vi "realtime_trans.vi"() -> ()   [LabVIEW 2015]
uses:
  <vilib>/rvi/interface/nirviOpenFPGA/nirviOpenFPGA.xnode
  <vilib>/rvi/interface/nirviReadWriteControl/nirviReadWriteControl.xnode
  <vilib>/Instr/_visa.llb/VISA Configure Serial Port (Instr).vi
  FPGA/FPGA_Transmission.vi
  <vilib>/functionblocks/FB Core/FB Core.xnode
  <vilib>/functionblocks/Control/PID/PID.vi
  <vilib>/functionblocks/NI_FunctionBlock Libraries.lvlib
  NiFpgaLv.dll
  <vilib>/Utility/error.llb/Error Cluster From Error Code.vi
  <vilib>/rvi/errors/niLvFpgaAdjustHostInterfaceError.vi
  FPGA Bitfiles/Controlsoftware2_FPGATarget4_FPGATransmission_apjjT0zB-SU.lvbitx
  <vilib>/FPGAPlugInAG/cRIO-9074/niLvFpga_Open_cRIO-9074.vi
panel:
  in  "Tab Control":enum32{"control", "Junk"}(tab)
  out "Steerer X+":dbl
  out "Steerer X-":dbl
  out "Steerer Y+":dbl
  out "Steerer Y-":dbl
  out "ExB +":dbl
  out "ExB -":dbl
  out "X+ V":fxp<+/-,26,5> format="%.23g"
  out "X+ I":fxp<+/-,26,5> format="%_4g"
  out "X- V":fxp<+/-,26,5> format="%_4g"
  out "X-I":fxp<+/-,26,5> format="%_4g"
  out "Y+ V":fxp<+/-,26,5> format="%_4g"
  out "Y+I":fxp<+/-,26,5> format="%_4g"
  out "Y-V":fxp<+/-,26,5> format="%_4g"
  out "Y-I":fxp<+/-,26,5> format="%_4g"
  out "ExB + V":fxp<+/-,26,5> format="%_4g"
  out "ExB +I":fxp<+/-,26,5> format="%_4g"
  out "ExB -V":fxp<+/-,26,5> format="%_4g"
  out "ExB-I":fxp<+/-,26,5> format="%_4g"
  out "concatenated string":string
  out "Ion gauge switch object cluser 2":T1
  out "Ion gauge anal waist Cluster 1":T1
  out "EXB":dbl
  in  "derivative time (Td, min)":dbl=0.05
  in  "integral time (Ti, min)":dbl=0.01
  in  "proportional gain (Kc)":dbl=25.0
  out "concatenated string 2":string
  out "anal field read":dbl
  out "unsigned byte array":u8[](array[numeric])
  out "Analyze read":u8[](array[numeric])
  out "analyze magnet set field":dbl
  out "element":dbl
  in  "diverter":bool
  out "diverter":bool
  out "error out":errorcluster
  out "error out 3":errorcluster
  out "error out 2":errorcluster
  in  "Ion gauge cluster control":T1
  out "Convectron 3":u8[](array[numeric])
  out "Ion gauge 4":u8[](array[numeric])
  out "Convectron 4":u8[](array[numeric])
  out "Ion gauge 5":u8[](array[numeric])
  out "Convectron 2":u8[](array[numeric])
  out "Ion gauge 2":u8[](array[numeric])
  out "Convectron 1":u8[](array[numeric])
  out "Ion gauge 1":u8[](array[numeric])
  out "error out 4":errorcluster
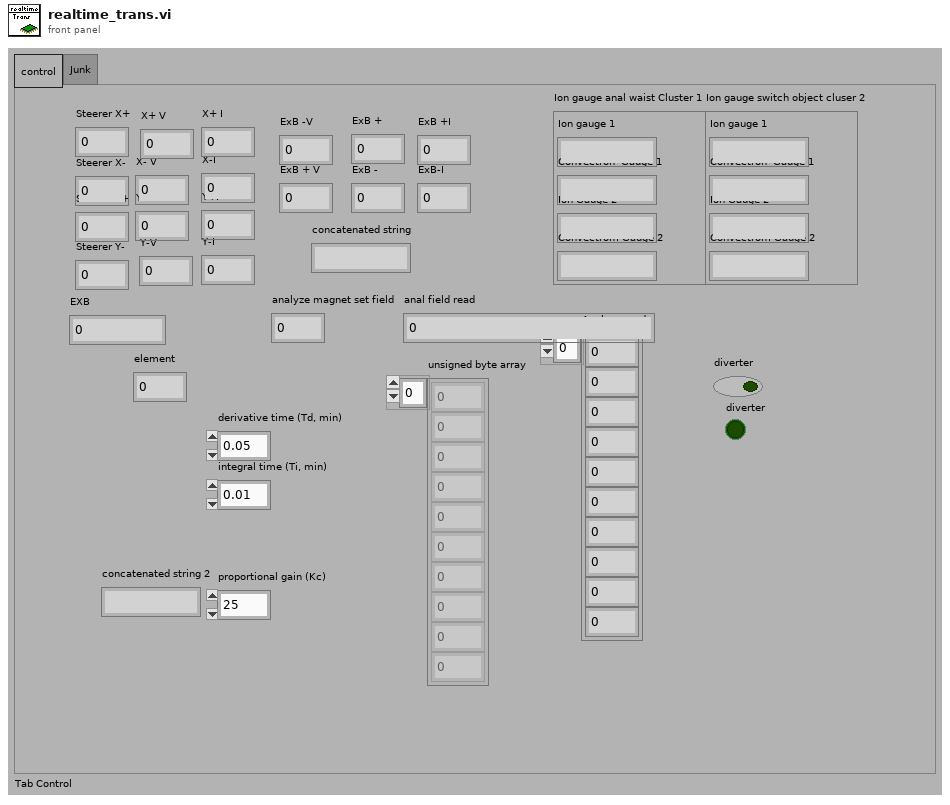
[diagram p1: front panel]
types:
  T1 = cluster{"Ion gauge 1":string, "Convectron  Gauge 1 ":string, "Ion Gauge 2":string, "Convectrom Gauge 2":string}
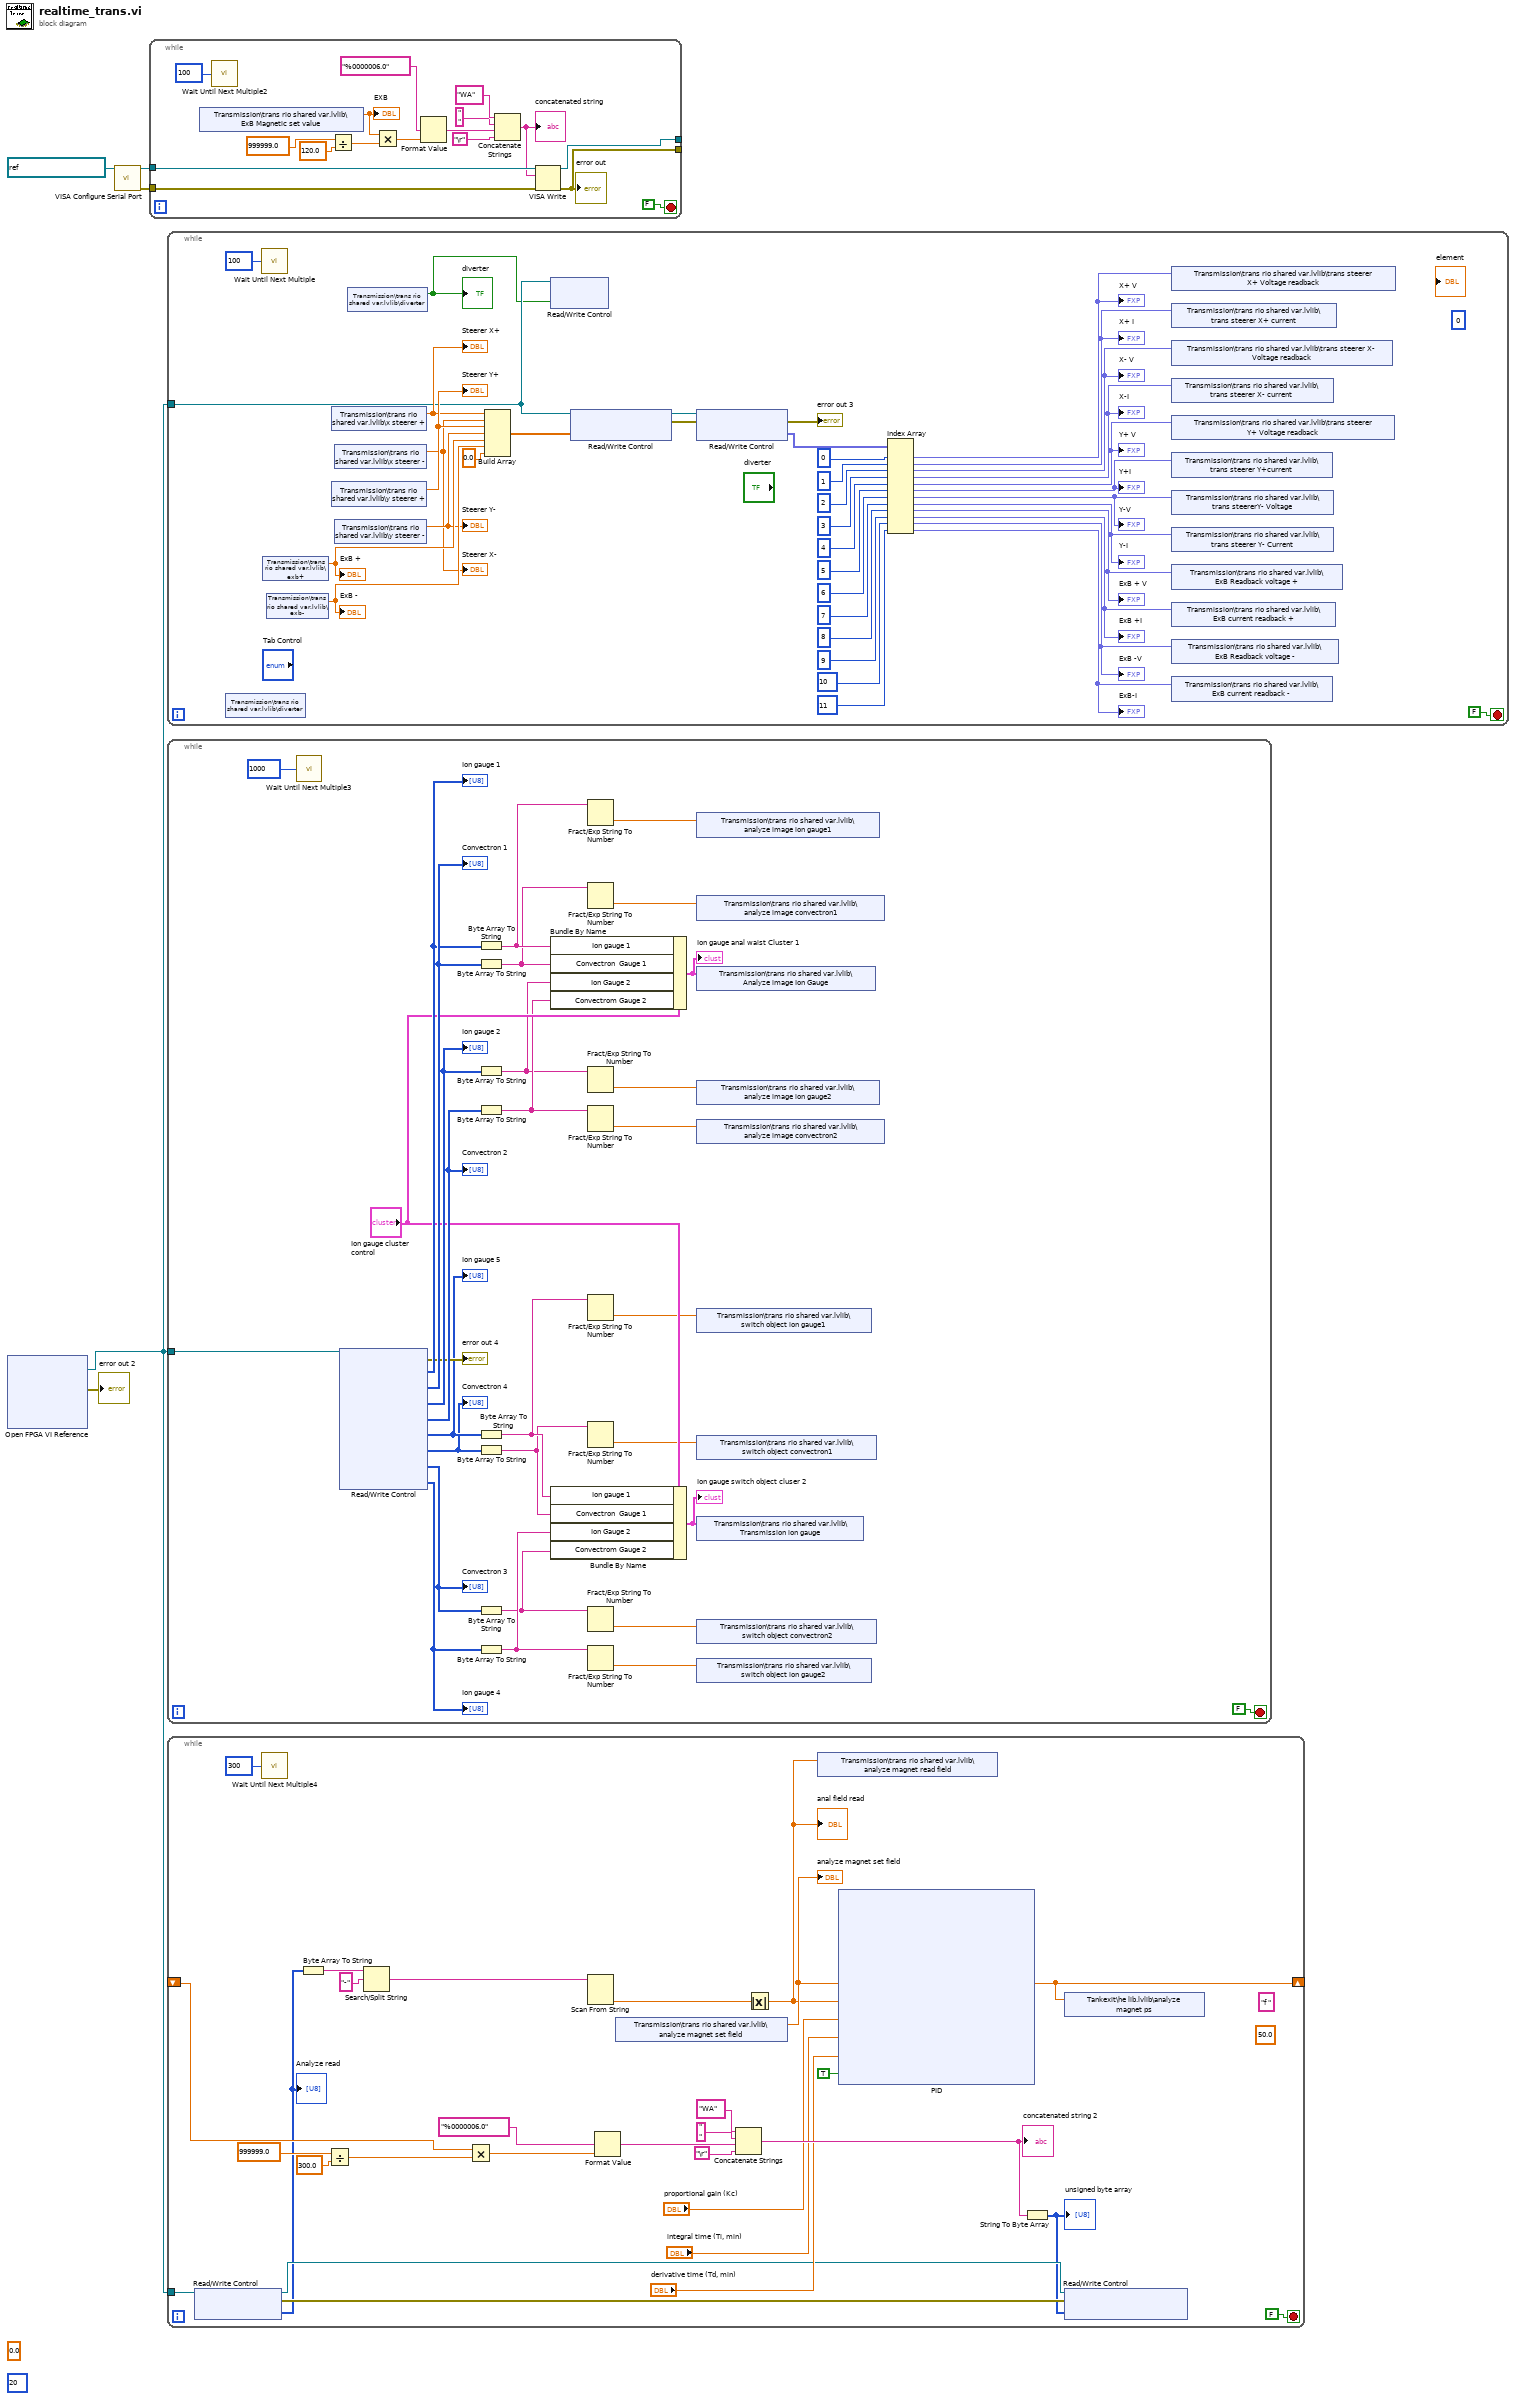
[diagram p0: block diagram]
diagram:
  (unwired) 20 ("dimension size")
  (unwired) 0.0 ("output")
  n1 = xnode "Open FPGA VI Reference"() -> ("FPGA VI Reference Out"=w1:refnum<k20>, "error out"=→"error out 2":errorcluster)  [unwired: 2 in]
  n2 = call-poly "VISA Configure Serial Port"("VISA resource name"=refnum<visa-resource-name> "ASRL1::INSTR") -> ("VISA resource name out"=w5:refnum<visa-resource-name>, "error out"=w4:errorcluster)  [unwired: 5 in, 8 out]
  n3 = while {
    tunnel: w4 -> [w12]
    tunnel: w5 -> [w11]
    tunnel: [w9] -> _
    tunnel: [w8] -> _
    stop <- FALSE stop-if-true
    n4 = shared-variable "Transmission\\trans rio shared var.lvlib\\ExB Magnetic set value"() -> (w7:dbl)  [unwired: 1 in, 1 out]
    "EXB" <- w7
    n5 = call "Wait Until Next Multiple2"("Count(mSec)"=u32 100) -> ()  [unwired: 1 out]
    n6 = Divide(x=999999.0, y=120.0) -> (x/y=w20:dbl)
    n7 = Multiply(x=w7, y=w20) -> (x*y=w13:dbl)
    n8 = Format Value(format string="%0000006.0", value (0)=w13) -> (output string=w16:string)  [unwired: 1 out]
    n9 = Concatenate Strings("WA", " ", w16, "\r") -> (w10:string)
    "concatenated string" <- w10
    n10 = VISA Write(VISA resource name=w11, write buffer=w10, error in (no error)=w12) -> (VISA resource name out=w9:refnum<visa-resource-name>, error out=w8:errorcluster)  [unwired: 1 out]
    "error out" <- w8
  }
  n11 = while {
    tunnel: w1 -> [w24]
    stop <- FALSE stop-if-true
    (unwired) 0 ("dimension size")
    n12 = shared-variable "Transmission\\trans rio shared var.lvlib\\diverter"() -> ()  [unwired: 1 in, 2 out]
    n13 = call "Wait Until Next Multiple"("Count(mSec)"=u32 100) -> ()  [unwired: 1 out]
    n14 = shared-variable "Transmission\\trans rio shared var.lvlib\\exb+"() -> (w47:dbl)  [unwired: 1 in, 1 out]
    "ExB +" <- w47
    n15 = shared-variable "Transmission\\trans rio shared var.lvlib\\exb-"() -> (w48:dbl)  [unwired: 1 in, 1 out]
    "ExB -" <- w48
    n16 = shared-variable "Transmission\\trans rio shared var.lvlib\\x steerer +"() -> (w43:dbl)  [unwired: 1 in, 1 out]
    "Steerer X+" <- w43
    n17 = shared-variable "Transmission\\trans rio shared var.lvlib\\y steerer +"() -> (w45:dbl)  [unwired: 1 in, 1 out]
    "Steerer Y+" <- w45
    n18 = shared-variable "Transmission\\trans rio shared var.lvlib\\x steerer -"() -> (w44:dbl)  [unwired: 1 in, 1 out]
    "Steerer X-" <- w44
    n19 = shared-variable "Transmission\\trans rio shared var.lvlib\\y steerer -"() -> (w46:dbl)  [unwired: 1 in, 1 out]
    "Steerer Y-" <- w46
    n20 = shared-variable "Transmission\\trans rio shared var.lvlib\\diverter"() -> (w23:bool)  [unwired: 1 in, 1 out]
    "diverter" <- w23
    n21 = Build Array(w43, w44, w45, w46, w47, w48, 0.0 ("element")) -> (w62:dbl[])
    n22 = xnode "Read/Write Control"("FPGA VI Reference In"=w24, "diverter"=w23) -> ()  [unwired: 1 in, 2 out]
    n23 = xnode "Read/Write Control"("FPGA VI Reference In"=w24, "Analog Output"=w62) -> ("FPGA VI Reference Out"=w28:refnum<k20>, "error out"=w27:errorcluster)  [unwired: 1 in]
    n24 = xnode "Read/Write Control"("FPGA VI Reference In"=w28, "error in"=w27) -> ("error out"=→"error out 3":errorcluster, "Analog input"=w29:fxp<+/-,26,5>[])  [unwired: 1 out]
    n25 = Index Array(array=w29, index #1=0 ("index"), index #2=1 ("index"), index #3=2 ("index"), index #4=3 ("index"), index #5=4 ("index"), index #6=5 ("index"), index #7=6 ("index"), index #8=7 ("index"), index #9=8 ("index"), index #10=9 ("index"), index #11=10 ("index"), index #12=11 ("index")) -> (element #1=w41:fxp<+/-,26,5>, element #2=w39:fxp<+/-,26,5>, element #3=w40:fxp<+/-,26,5>, element #4=w42:fxp<+/-,26,5>, element #5=w38:fxp<+/-,26,5>, element #6=w36:fxp<+/-,26,5>, element #7=w37:fxp<+/-,26,5>, element #8=w35:fxp<+/-,26,5>, element #9=w34:fxp<+/-,26,5>, element #10=w32:fxp<+/-,26,5>, element #11=w33:fxp<+/-,26,5>, element #12=w31:fxp<+/-,26,5>)
    "X+ V" <- w41
    "X+ I" <- w39
    "X- V" <- w40
    "X-I" <- w42
    "Y+ V" <- w38
    "Y+I" <- w36
    "Y-V" <- w37
    "Y-I" <- w35
    "ExB + V" <- w34
    "ExB +I" <- w32
    "ExB -V" <- w33
    "ExB-I" <- w31
    n26 = shared-variable "Transmission\\trans rio shared var.lvlib\\trans steerer X+ Voltage readback"(w41) -> ()  [unwired: 1 in, 1 out]
    n27 = shared-variable "Transmission\\trans rio shared var.lvlib\\trans steerer X+ current"(w39) -> ()  [unwired: 1 in, 1 out]
    n28 = shared-variable "Transmission\\trans rio shared var.lvlib\\trans steerer X- Voltage readback"(w40) -> ()  [unwired: 1 in, 1 out]
    n29 = shared-variable "Transmission\\trans rio shared var.lvlib\\trans steerer X- current"(w42) -> ()  [unwired: 1 in, 1 out]
    n30 = shared-variable "Transmission\\trans rio shared var.lvlib\\trans steerer Y+ Voltage readback"(w38) -> ()  [unwired: 1 in, 1 out]
    n31 = shared-variable "Transmission\\trans rio shared var.lvlib\\trans steerer Y+current"(w36) -> ()  [unwired: 1 in, 1 out]
    n32 = shared-variable "Transmission\\trans rio shared var.lvlib\\trans steererY- Voltage"(w37) -> ()  [unwired: 1 in, 1 out]
    n33 = shared-variable "Transmission\\trans rio shared var.lvlib\\trans steerer Y- Current"(w35) -> ()  [unwired: 1 in, 1 out]
    n34 = shared-variable "Transmission\\trans rio shared var.lvlib\\ExB Readback voltage +"(w34) -> ()  [unwired: 1 in, 1 out]
    n35 = shared-variable "Transmission\\trans rio shared var.lvlib\\ExB current readback +"(w32) -> ()  [unwired: 1 in, 1 out]
    n36 = shared-variable "Transmission\\trans rio shared var.lvlib\\ExB Readback voltage -"(w33) -> ()  [unwired: 1 in, 1 out]
    n37 = shared-variable "Transmission\\trans rio shared var.lvlib\\ExB current readback -"(w31) -> ()  [unwired: 1 in, 1 out]
  }
  n38 = while {
    tunnel: w1 -> [w81]
    stop <- FALSE stop-if-true
    n39 = call "Wait Until Next Multiple3"("Count(mSec)"=u32 1000 ("millisecond multiple")) -> ()  [unwired: 1 out]
    n40 = xnode "Read/Write Control"("FPGA VI Reference In"=w81) -> ("error out"=→"error out 4":errorcluster, "Ion gauge 1"=w90:u8[], "Convectron 1"=w91:u8[], "Ion gauge 2"=w92:u8[], "Convectron 2"=w93:u8[], "Ion gauge 3"=w87:u8[], "Convectron 3"=w86:u8[], "Convectron 4"=w84:u8[], "Ion gauge 4"=w85:u8[])  [unwired: 1 in, 1 out]
    "Ion gauge 1" <- w90
    "Convectron 1" <- w91
    "Ion gauge 2" <- w92
    "Convectron 2" <- w93
    "Ion gauge 5" <- w87
    "Convectron 4" <- w86
    "Ion gauge 4" <- w85
    "Convectron 3" <- w84
    n41 = Byte Array To String(unsigned byte array=w90) -> (string=w70:string)
    n42 = Byte Array To String(unsigned byte array=w91) -> (string=w69:string)
    n43 = Byte Array To String(unsigned byte array=w92) -> (string=w67:string)
    n44 = Byte Array To String(unsigned byte array=w93) -> (string=w68:string)
    n45 = Byte Array To String(unsigned byte array=w87) -> (string=w78:string)
    n46 = Byte Array To String(unsigned byte array=w86) -> (string=w77:string)
    n47 = Byte Array To String(unsigned byte array=w84) -> (string=w75:string)
    n48 = Byte Array To String(unsigned byte array=w85) -> (string=w76:string)
    n49 = Bundle By Name(cluster="Ion gauge cluster control", "Ion gauge 1"=w70, "Convectron  Gauge 1"=w69, "Ion Gauge 2"=w67, "Convectrom Gauge 2"=w68) -> (w79:T1)
    "Ion gauge anal waist Cluster 1" <- w79
    n50 = Bundle By Name(cluster="Ion gauge cluster control", "Ion gauge 1"=w78, "Convectron  Gauge 1"=w77, "Ion Gauge 2"=w76, "Convectrom Gauge 2"=w75) -> (w80:T1)
    "Ion gauge switch object cluser 2" <- w80
    n51 = Fract/Exp String To Number(string=w70) -> (number=w66:dbl)  [unwired: 3 in, 1 out]
    n52 = Fract/Exp String To Number(string=w69) -> (number=w64:dbl)  [unwired: 3 in, 1 out]
    n53 = Fract/Exp String To Number(string=w67) -> (number=w65:dbl)  [unwired: 3 in, 1 out]
    n54 = Fract/Exp String To Number(string=w68) -> (number=w63:dbl)  [unwired: 3 in, 1 out]
    n55 = Fract/Exp String To Number(string=w78) -> (number=w74:dbl)  [unwired: 3 in, 1 out]
    n56 = Fract/Exp String To Number(string=w77) -> (number=w73:dbl)  [unwired: 3 in, 1 out]
    n57 = Fract/Exp String To Number(string=w75) -> (number=w71:dbl)  [unwired: 3 in, 1 out]
    n58 = Fract/Exp String To Number(string=w76) -> (number=w72:dbl)  [unwired: 3 in, 1 out]
    n59 = shared-variable "Transmission\\trans rio shared var.lvlib\\analyze image ion gauge1"(w66) -> ()  [unwired: 1 in, 1 out]
    n60 = shared-variable "Transmission\\trans rio shared var.lvlib\\analyze image convectron1"(w64) -> ()  [unwired: 1 in, 1 out]
    n61 = shared-variable "Transmission\\trans rio shared var.lvlib\\Analyze image Ion Gauge"(w79) -> ()  [unwired: 1 in, 1 out]
    n62 = shared-variable "Transmission\\trans rio shared var.lvlib\\analyze image ion gauge2"(w65) -> ()  [unwired: 1 in, 1 out]
    n63 = shared-variable "Transmission\\trans rio shared var.lvlib\\analyze image convectron2"(w63) -> ()  [unwired: 1 in, 1 out]
    n64 = shared-variable "Transmission\\trans rio shared var.lvlib\\switch object ion gauge1"(w74) -> ()  [unwired: 1 in, 1 out]
    n65 = shared-variable "Transmission\\trans rio shared var.lvlib\\switch object convectron1"(w73) -> ()  [unwired: 1 in, 1 out]
    n66 = shared-variable "Transmission\\trans rio shared var.lvlib\\Transmission ion gauge"(w80) -> ()  [unwired: 1 in, 1 out]
    n67 = shared-variable "Transmission\\trans rio shared var.lvlib\\switch object convectron2"(w71) -> ()  [unwired: 1 in, 1 out]
    n68 = shared-variable "Transmission\\trans rio shared var.lvlib\\switch object ion gauge2"(w72) -> ()  [unwired: 1 in, 1 out]
  }
  n69 = while {
    shift-right: [w108] -> _
    shift-left: _ -> [w97]
    tunnel: w1 -> [w102]
    stop <- FALSE stop-if-true
    (unwired) 50.0 ("x")
    (unwired) "f " ("regular expression")
    n70 = xnode "Read/Write Control"("FPGA VI Reference In"=w102) -> ("FPGA VI Reference Out"=w101:refnum<k20>, "error out"=w100:errorcluster, "Analyze read"=w96:u8[])  [unwired: 1 in]
    "Analyze read" <- w96
    n71 = call "Wait Until Next Multiple4"("Count(mSec)"=u32 300 ("millisecond multiple")) -> ()  [unwired: 1 out]
    n72 = Byte Array To String(unsigned byte array=w96) -> (string=w110:string)
    n73 = Divide(x=999999.0, y=300.0) -> (x/y=w115:dbl)
    n74 = Search/Split String(string=w110, search string/char (-)="-") -> (match + rest of string=w98:string)  [unwired: 3 out]
    n75 = Multiply(x=w97, y=w115) -> (x*y=w117:dbl)
    n76 = Scan From String(input string=w98) -> (output 1=w109:dbl)  [unwired: 3 in, 4 out]
    n77 = Format Value(format string="%0000006.0", value (0)=w117) -> (output string=w120:string)  [unwired: 1 out]
    n78 = shared-variable "Transmission\\trans rio shared var.lvlib\\analyze magnet set field"() -> (w95:dbl)  [unwired: 1 in, 1 out]
    "analyze magnet set field" <- w95
    n79 = Concatenate Strings("WA", " ", w120, "\r") -> (w121:string)
    "concatenated string 2" <- w121
    n80 = Absolute Value(x=w109) -> (abs(x)=w94:dbl)
    "anal field read" <- w94
    n81 = shared-variable "Transmission\\trans rio shared var.lvlib\\analyze magnet read field"(w94) -> ()  [unwired: 1 in, 1 out]
    n82 = xnode "PID"("setpoint"=w95, "process variable"=w94, "proportional gain (Kc)"="proportional gain (Kc)", "integral time (Ti, min)"="integral time (Ti, min)", "derivative time (Td, min)"="derivative time (Td, min)", "auto? (T)"=TRUE) -> ("output"=w108:dbl)  [unwired: 1 in, 1 out]
    n83 = String To Byte Array(string=w121) -> (unsigned byte array=w99:u8[])
    "unsigned byte array" <- w99
    n84 = shared-variable "Tankexit\\he lib.lvlib\\analyze magnet ps"(w108) -> ()  [unwired: 1 in, 1 out]
    n85 = xnode "Read/Write Control"("FPGA VI Reference In"=w101, "error in"=w100, "analyze ps set array"=w99) -> ()  [unwired: 2 out]
  }
